vi "Ventaneo.vi"() -> ()   [LabVIEW 2018]
uses:
  <vilib>/imath/engines/lvmath2/RunTimeEngine/BuiltInFunctions/fir_win/NIMS_fir_win(I32,V,Str,V,Str).vi
  <vilib>/imath/engines/lvmath2/RunTimeEngine/ErrorHandling/NIMS_Create Error From Enums.vi
  <vilib>/imath/engines/lvmath2/RunTimeEngine/BuiltInFunctions/figure/NIMS_figure(I32).vi
  <vilib>/imathl/engines/lvmath/Functions/Error Handling/Create Error.vi
  <vilib>/imath/engines/lvmath2/RunTimeEngine/BuiltInFunctions/plot/NIMS_plot(G, Str).vi
  <instcachedir>/0/NIMS_plot(G, Str)_F55567436FC345288A9397CFB037001B.lvgen/NIMS_plot(G, Str)_F55567436FC345288A9397CFB037001B_000.vi
  <vilib>/imath/engines/lvmath2/RunTimeEngine/BuiltInFunctions/freqzd/NIMS_NoOutput_freqzd().vi
  <vilib>/imath/engines/lvmath2/RunTimeEngine/NodeEndStatement/NIMS_NodeEndStatement_Output.vi
  <instcachedir>/0/NIMS_NodeEndStatement_Output_53EC0D466D134D7ABD903AC30B43404B.lvgen/NIMS_NodeEndStatement_Output_53EC0D466D134D7ABD903AC30B43404B_005.vi
  <vilib>/imath/engines/lvmath2/RunTimeEngine/ErrorHandling/NIMS_Finalize Error.vi
panel:
  in  "stop":bool
  out "Array":dbl[](array[numeric])
  in  "ventana 5":bool
  in  "ventana 4":bool
  in  "ventana 3":bool
  in  "ventana 2":bool
  in  "ventana 1":bool
  in  "Fs":dbl
  in  "n":dbl
  in  "wn":dbl
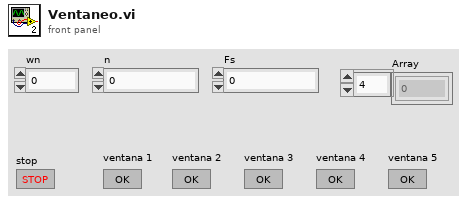
[diagram p1: front panel]
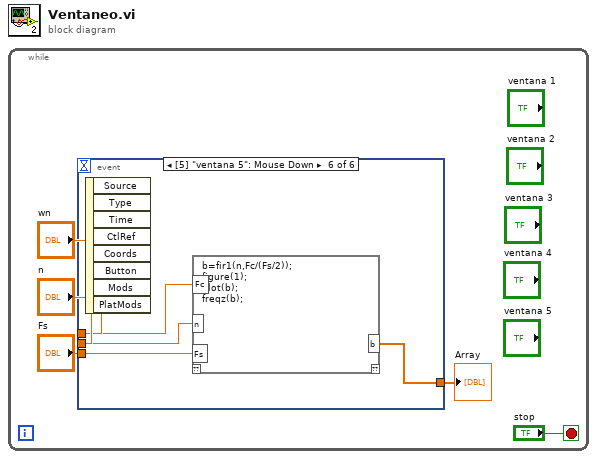
[diagram p0: block diagram]
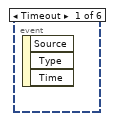
[diagram p2: hidden frame]
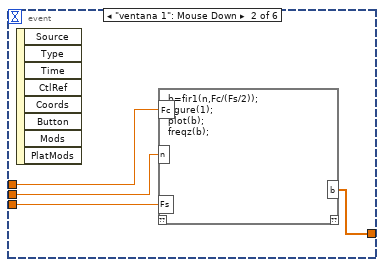
[diagram p3: hidden frame]
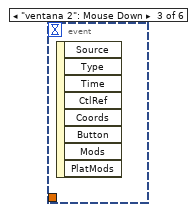
[diagram p4: hidden frame]
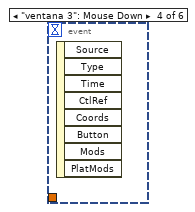
[diagram p5: hidden frame]
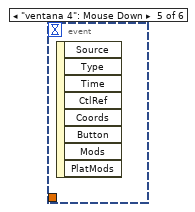
[diagram p6: hidden frame]
diagram:
  n1 = while {
    stop <- "stop" stop-if-true
    n2 = event shown="[5] \"ventana 5\": Mouse Down" {
      selector: _ -> [_ _ _ _ _ _]
      dyn-events: _ -> [_ _ _ _ _ _]
      timeout: _ -> [_ _ _ _ _ _]
      tunnel: [_ w9 _ _ _ w104] -> w5
      tunnel: "Fs" -> [_ w8 _ _ _ w107]
      tunnel: "n" -> [_ w7 _ _ _ w106]
      tunnel: "wn" -> [_ w6 _ _ _ w105]
      event Timeout {
        n3 = event-data() -> ()  [unwired: 1 in, 3 out]
      }
      event "ventana 1": Mouse Down {
        n4 = event-data() -> ()  [unwired: 1 in, 8 out]
        n5 = mathscript code="b=fir1(n,Fc/(Fs/2));\nfigure(1);\nplot(b);\nfreqz(b);"("n"=w7, "Fc"=w6, "Fs"=w8) -> ("b"=w9:dbl[])  [unwired: 1 in, 1 out]
      }
      event "ventana 2": Mouse Down {
        n6 = event-data() -> ()  [unwired: 1 in, 8 out]
      }
      event "ventana 3": Mouse Down {
        n7 = event-data() -> ()  [unwired: 1 in, 8 out]
      }
      event "ventana 4": Mouse Down {
        n8 = event-data() -> ()  [unwired: 1 in, 8 out]
      }
      event "ventana 5": Mouse Down {
        n9 = event-data() -> ()  [unwired: 1 in, 8 out]
        n10 = mathscript code="b=fir1(n,Fc/(Fs/2));\nfigure(1);\nplot(b);\nfreqz(b);"("n"=w106, "Fc"=w105, "Fs"=w107) -> ("b"=w104:dbl[])  [unwired: 1 in, 1 out]
      }
    }
    "Array" <- w5
  }
